vi "getRef.vi"(8 "error in (no error)":errorcluster) -> (0 "error out":errorcluster, 2 "partstracking_controller_ref":refnum<class "PartsTracking Controller.lvclass">)   [LabVIEW 2014, in "PartsTracking Controller.lvclass"]
uses:
  PartsTracking Controller.lvclass
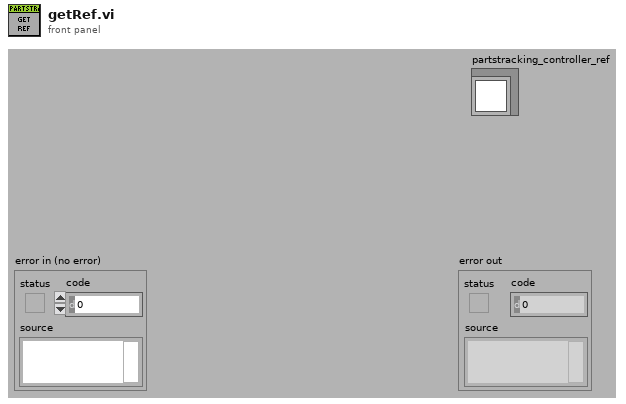
[diagram p1: front panel]
types:
  T1 = typedef "PartsTracking Controller.lvclass/ClassAttributesRef.ctl" = refnum<data-value>
  T2 = typedef "PartsTracking Controller.lvclass/ClassAttributes.ctl" = cluster{"Dummy":bool, "partstracking_controller_ref":refnum<class "PartsTracking Controller.lvclass">}
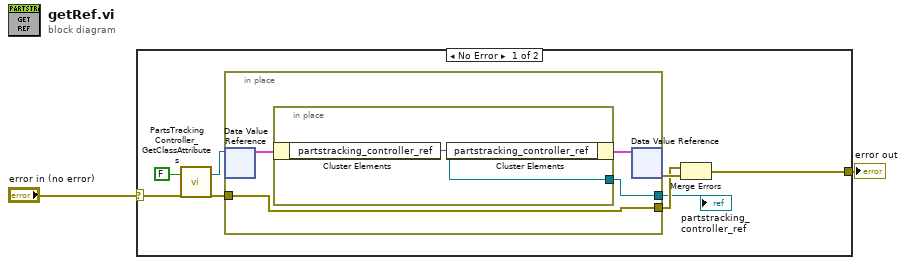
[diagram p0: block diagram]
diagram:
  n1 = case shown="No Error" "error in (no error)" {
    selector: "error in (no error)" -> [w6 w16]
    tunnel: [w10 w16] -> w1
    frame No Error {
      n2 = call "PartsTracking Controller_GetClassAttributes.vi"("return data? (T)"=FALSE, "error in (no error)"=w6) -> ("class attributes ref"=w4:T1, "error out"=w5:errorcluster)  [unwired: 14 in, 2 out]
      n3 = in-place {
        in-place-border: w5 -> [w12]
        in-place-border: [w12] -> w8
        in-place-border: [w11] -> w3
        n4 = in-place-dvr #1(w4) -> (w13:T2)  [unwired: 1 out]
        n5 = in-place {
          in-place-border: [w15] -> w11
          n6 = in-place-cluster #2(w13) -> ("partstracking_controller_ref"=w15:refnum<class "PartsTracking Controller.lvclass">)
          n7 = in-place-cluster #2("partstracking_controller_ref"=w15) -> (w14:T2)
        }
        n8 = in-place-dvr #1(w14) -> (w9:errorcluster)  [unwired: 1 out]
      }
      "partstracking_controller_ref" <- w3
      n9 = Merge Errors(w8, w9) -> (w10:errorcluster)
    }
    frame Error {
    }
  }
  "error out" <- w1
